vi "Decorate And Unified Msg Set.vi"(9 "Persistent Layers":refnum<class "Actor.lvclass">[](array[class]), 10 "Local Layers":refnum<class "Actor.lvclass">[](array[class])) -> (1 "Unified Msg Set":T1, 2 "Unified Actor":refnum<class "Actor.lvclass">)   [LabVIEW 2025, in "jettl.lvlib"]
uses:
  jettl.lvlib
  Actor/Actor.lvclass
  Msg Set.ctl
  Msg/Msg.lvclass
  Core Actor/Core Actor.lvlib
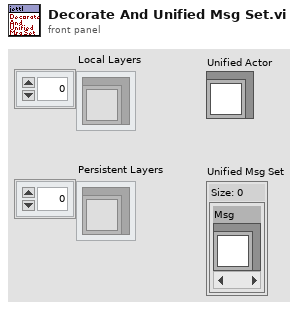
[diagram p1: front panel]
types:
  T1 = typedef "jettl.lvlib/Msg Set.ctl" = set{refnum<class "Msg.lvclass">}
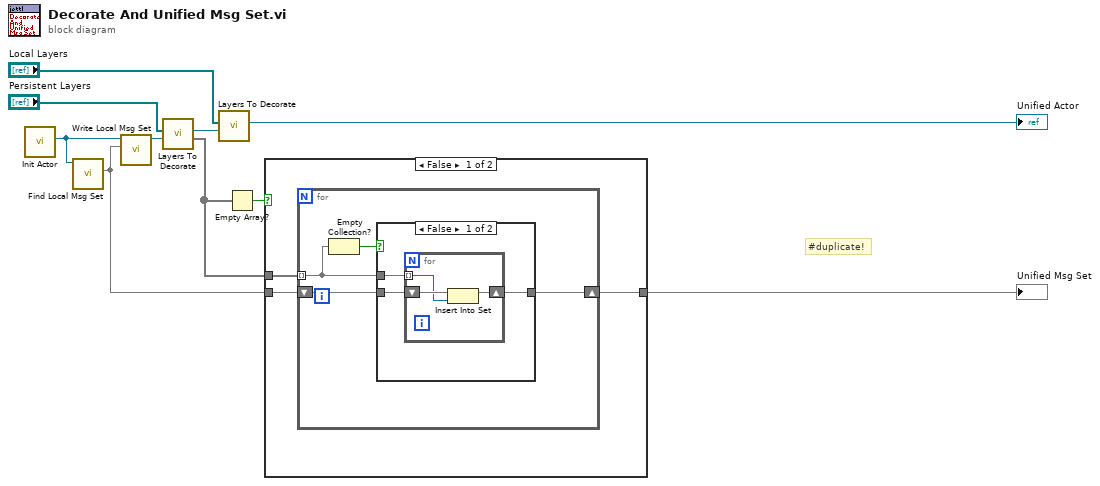
[diagram p0: block diagram]
diagram:
  # "#duplicate!"
  n1 = call "Init Actor.vi"() -> ("Actor"=w6:refnum<class "Actor.lvclass">)  [unwired: 11 in]
  n2 = call-dynamic "Find Local Msg Set.vi"("Actor in"=w6) -> ("Local Msg Set"=w5:T1)  [unwired: 10 in]
  n3 = call-dynamic "Write Local Msg Set.vi"("Local Msg Set"=w5, "Actor in"=w6) -> ("Actor out"=w4:refnum<class "Actor.lvclass">)  [unwired: 9 in]
  n4 = call "Layers To Decorate.vi"("Actor To Decorate"=w4, "Layers"="Persistent Layers") -> ("Local Msg Sets"=w3:T1[], "Decorated Actor"=w10:refnum<class "Actor.lvclass">)  [unwired: 8 in]
  n5 = call "Layers To Decorate.vi"("Actor To Decorate"=w10, "Layers"="Local Layers") -> ("Decorated Actor"=→"Unified Actor":refnum<class "Actor.lvclass">)  [unwired: 8 in, 1 out]
  n6 = Empty Array?(array=w3) -> (empty?=w2:bool)
  n7 = case shown="False" w2 {
    tunnel: w3 -> [w13 _]
    tunnel: w5 -> [w12 w25]
    tunnel: [w11 w25] -> w1
    frame False {
      n8 = for {
        tunnel: w13 -> [w15] mode=indexing
        shift-right: [w16] -> w11
        shift-left: w12 -> [w17]
        n9 = Empty Collection?(1:w15) -> (0:w14:bool)
        n10 = case shown="False" w14 {
          tunnel: w17 -> [w20 w24]
          tunnel: [w19 w24] -> w16
          tunnel: w15 -> [w18 _]
          frame False {
            n11 = for {
              shift-right: [w22] -> w19
              shift-left: w20 -> [w23]
              tunnel: w18 -> [w21] mode=indexing
              n12 = Insert Into Set(10:w21, 11:w23) -> (3:w22:T1)  [unwired: 1 out]
            }
          }
          frame True {
          }
        }
      }
    }
    frame True {
    }
  }
  "Unified Msg Set" <- w1
